vi "Choreo_SwerveSample_OffsetBy.vi"(9 "TimeStampOffset":dbl, 11 "ChoreoSwerveSample":T1) -> (3 "OffsetSample":T1)   [LabVIEW 2019, in "ChoreoLib.lvlib"]
doc: "Returns this sample, offset by the given timestamp.\n \nInputs: \n -- ChoreoSwerveSample - cluster - Swerve sample.\n -- timestampOffset -- double - The offset to apply to the timestamp. (seconds)\n\nOutputs: \n -- OffsetSample - cluster - this sample, offset by the given timestamp."
uses:
  ChoreoLib.lvlib
  TypeDef/ChoreoSwerveSample.ctl
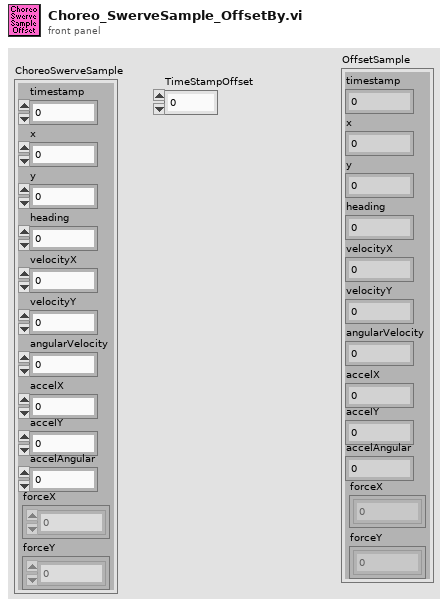
[diagram p1: front panel]
types:
  T1 = typedef "ChoreoLib.lvlib/ChoreoSwerveSample.ctl" = cluster{"timestamp":dbl, "x":dbl, "y":dbl, "heading":dbl, "velocityX":dbl, "velocityY":dbl, "angularVelocity":dbl, "accelX":dbl, "accelY":dbl, "accelAngular":dbl, "forceX":dbl[], "forceY":dbl[]}
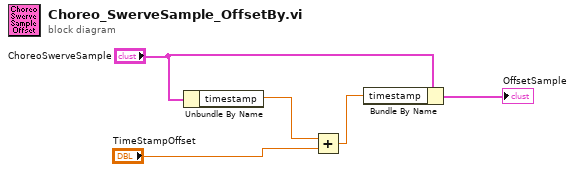
[diagram p0: block diagram]
diagram:
  n1 = Unbundle By Name("ChoreoSwerveSample") -> ("timestamp"=w2:dbl)
  n2 = Add(x=w2, y="TimeStampOffset") -> (x+y=w5:dbl)
  n3 = Bundle By Name(cluster="ChoreoSwerveSample", "timestamp"=w5) -> (→"OffsetSample":T1)
